vi "HSMS Start.vi"(8 "error in (no error)":errorcluster, 9 "Port":u16, 10 "IP Adrress":string, 11 "HSMS Class in":refnum<class "HSMS Class.lvclass">) -> (0 "error out":errorcluster, 3 "HSMS Class out":refnum<class "HSMS Class.lvclass">)   [LabVIEW 2020, in "SECS Communication.lvlib" / "HSMS Class.lvclass"]
uses:
  HSMS Class.lvclass
  HSMS Class.lvclass/HSMS Class.ctl
  Write Alive Notifier.vi
  Write Listener Refnum.vi
  Read HSMS State.vi
  Core.vi
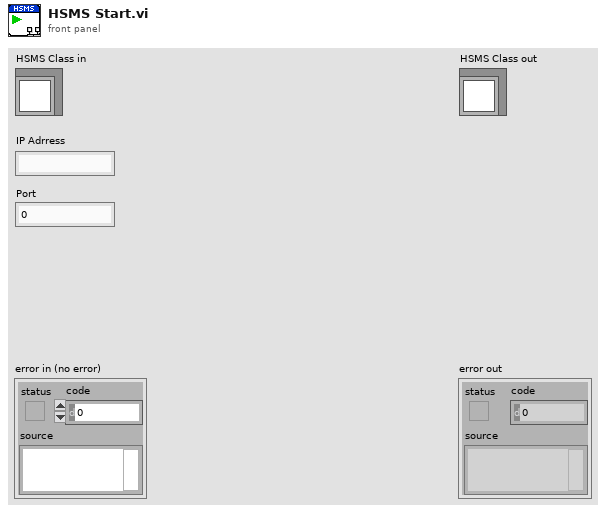
[diagram p1: front panel]
types:
  T1 = typedef "SECS Communication.lvlib/HSMS Class.lvclass/HSMS State.ctl" = enum16{"[TCP/IP]Not Connect", "[HSMS]Not Selected", "[HSMS]Selected", "Stop"}
  T2 = typedef "SECS Communication.lvlib/HSMS Class.lvclass/Role.ctl" = enum16{"Passive", "Active"}
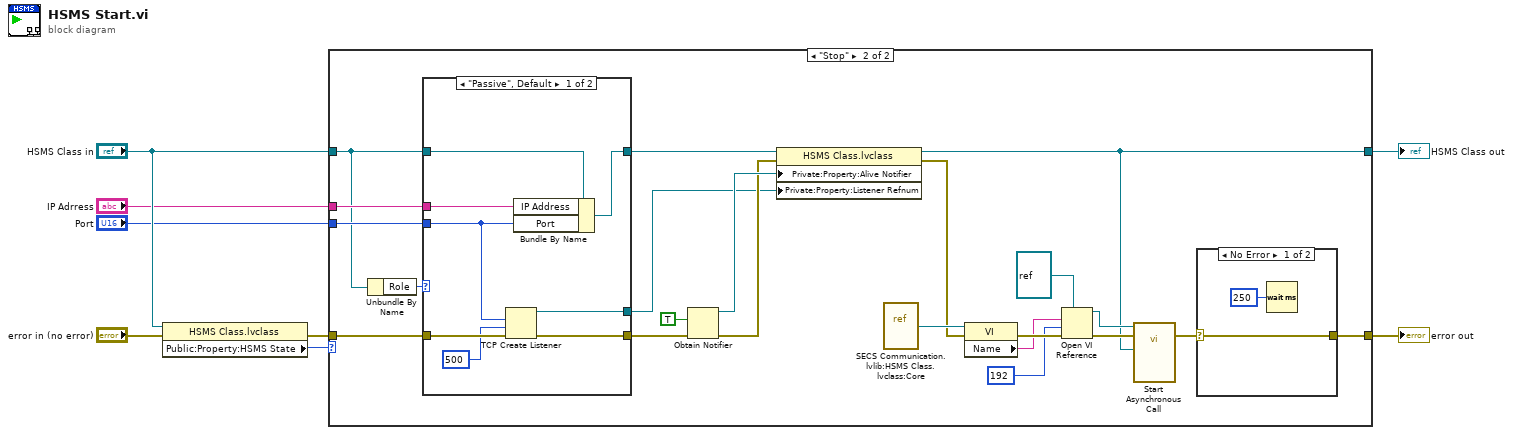
[diagram p0: block diagram]
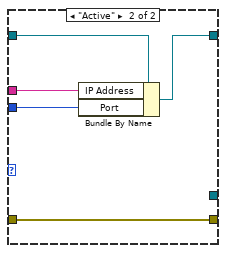
[diagram p3: hidden frame]
diagram:
  n1 = property class="HSMS Class.lvclass"(reference="HSMS Class in", error in="error in (no error)") -> (error out=w4:errorcluster, "Public:Property:HSMS State"=w3:T1)  [unwired: 1 out]
  n2 = case shown="\"Stop\"" w3 {
    tunnel: [w9 w24] -> w8
    tunnel: [w10 w12] -> w7
    tunnel: "HSMS Class in" -> [w10 w18]
    tunnel: w4 -> [w9 w22]
    tunnel: "IP Adrress" -> [_ w20]
    tunnel: "Port" -> [_ w19]
    frame Default {
    }
    frame "Stop" {
      n3 = Unbundle By Name(w18) -> ("Role"=w21:T2)
      n4 = case shown="\"Passive\", Default" w21 {
        tunnel: w22 -> [w40 w45]
        tunnel: w20 -> [w35 w43]
        tunnel: w19 -> [w34 w42]
        tunnel: w18 -> [w39 w44]
        tunnel: [w37 w41] -> w16
        tunnel: [w36 w45] -> w17
        tunnel: [w33 _] -> w11
        frame "Passive", Default {
          n5 = TCP Create Listener(8:w40, 9:500 ("timeout ms (25000)"), 10:w34) -> (0:w36:errorcluster, 3:w33:refnum<k5>)  [unwired: 2 in, 1 out]
          n6 = Bundle By Name(cluster=w39, "IP Address"=w35, "Port"=w34) -> (w37:refnum<class "HSMS Class.lvclass">)
        }
        frame "Active" {
          n7 = Bundle By Name(cluster=w44, "IP Address"=w43, "Port"=w42) -> (w41:refnum<class "HSMS Class.lvclass">)
        }
      }
      n8 = Obtain Notifier(notification data type=TRUE, error in (no error)=w17) -> (notifier out=w15:refnum<notifier>, error out=w14:errorcluster)  [unwired: 2 in, 1 out]
      n9 = property class="HSMS Class.lvclass"(reference=w16, error in=w14, "Private:Property:Alive Notifier"=w15, "Private:Property:Listener Refnum"=w11) -> (reference out=w12:refnum<class "HSMS Class.lvclass">, error out=w13:errorcluster)
      n10 = vi-ref "SECS Communication.lvlib:HSMS Class.lvclass:Core.vi"() -> (w32:refnum<vi>)
      n11 = property class="VI"(reference=w32, error in=w13) -> (error out=w31:errorcluster, "Name"=w30:string)  [unwired: 1 out]
      n12 = Open VI Reference(type specifier VI Refnum (for type only)=refnum<vi> refnum, vi path=w30, options=192, error in (no error)=w31) -> (vi reference=w26:refnum<vi>, error out=w27:errorcluster)  [unwired: 2 in]
      n13 = call-by-ref "Start Asynchronous Call"(reference=w26, error in=w27, "HSMS Class in"=w12) -> (error out=w25:errorcluster)  [unwired: 9 in, 3 out]
      n14 = case shown="No Error" w25 {
        selector: w25 -> [w47 w48]
        tunnel: [w47 w48] -> w24
        frame No Error {
          n15 = Wait (ms)(milliseconds to wait=u32 250) -> ()  [unwired: 1 out]
        }
        frame Error {
        }
      }
    }
  }
  "error out" <- w8
  "HSMS Class out" <- w7
